vi "Load Cryostat Class.vi"(8 "error in (no error)":errorcluster, 11 "SweepControl in":refnum<class "SweepControl.lvclass">) -> (0 "error out":errorcluster, 3 "SweepControl out":refnum<class "SweepControl.lvclass">)   [LabVIEW 2016]
uses:
  <userlib>/LevyLab/Levylab Instruments/Instrument Types/Cryostat/Instrument.Cryostat.lvclass
  Control Experiment/Control Experiment.lvclass
  SweepControl.lvclass
  C:/Program Files (x86)/National Instruments/LabVIEW 2016/vi.lib/JKI/JKI SMO/SMO/SMO.lvclass
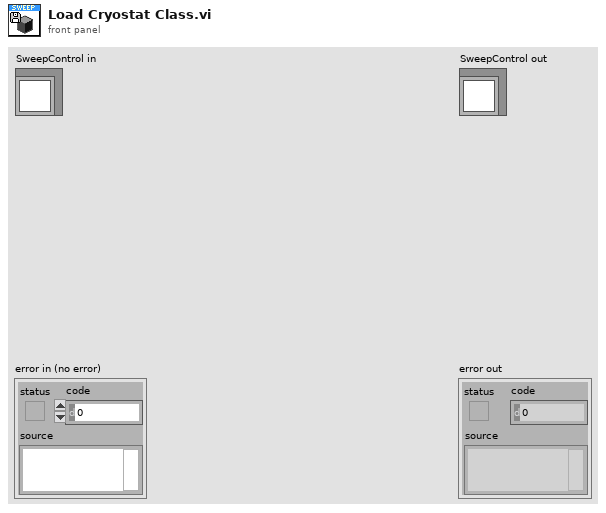
[diagram p1: front panel]
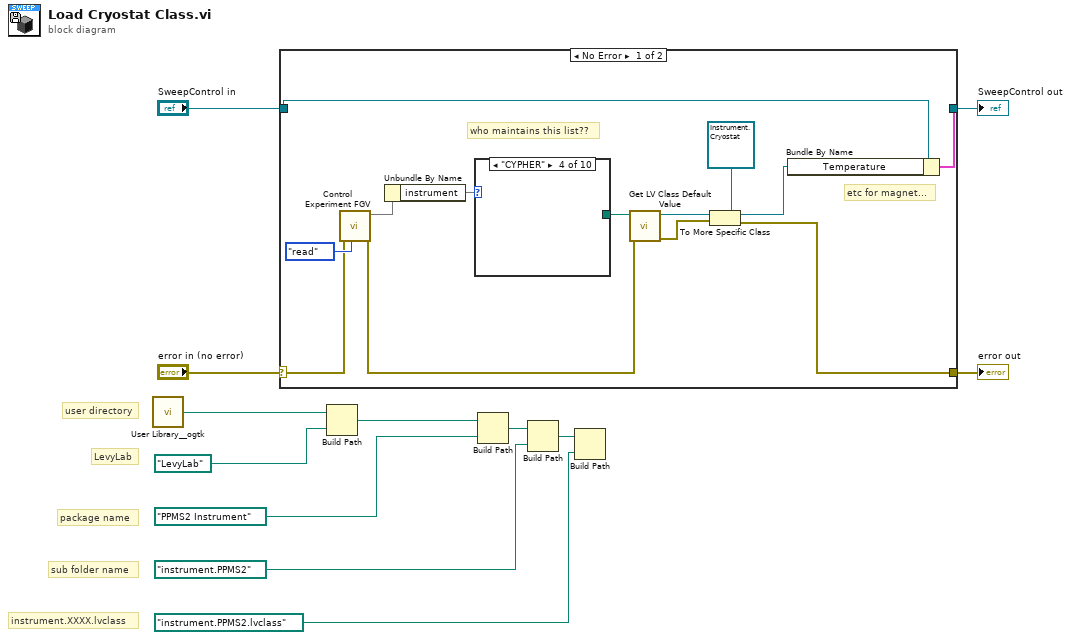
[diagram p0: block diagram]
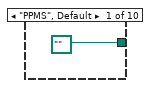
[diagram p2: hidden frame]
diagram:
  # "LevyLab"
  # "user directory"
  # "instrument.XXXX.lvclass"
  # "sub folder name"
  # "package name"
  n1 = call <userlib>:"User Library__ogtk.vi"() -> ("User Library (+ Relative)"=w8:path)  [unwired: 1 in]
  n2 = case shown="No Error" "error in (no error)" {
    selector: "error in (no error)" -> [w17 w28]
    tunnel: [w20 w28] -> w11
    tunnel: [w21 w27] -> w9
    tunnel: "SweepControl in" -> [w22 w27]
    frame No Error {
      # "who maintains this list??"
      # "etc for magnet..."
      n3 = call "Control Experiment FGV.vi"("Function"=enum16{"read", "write"}."read", "error in (no error)"=w17) -> ("error out"=w16:errorcluster, 2:w13)  [unwired: 7 in, 1 out]
      n4 = Unbundle By Name(w13) -> ("instrument"=w15)
      n5 = case shown="\"CYPHER\"" w15 {
        tunnel: [path "" ("class path") _ _ _ _ _ _ _ _ _] -> w14
        frame "PPMS", Default {
        }
        frame "PPMS2" {
        }
        frame "MFP3D" {
        }
        frame "CYPHER" {
        }
        frame "THz1" {
        }
        frame "THz2" {
        }
        frame "MNK" {
        }
        frame "CF900" {
        }
        frame "JEOL" {
        }
        frame "AGILENT" {
        }
      }
      n6 = call <vilib>:"Get LV Class Default Value.vi"("error in (no error)"=w16, "class path"=w14) -> ("error out"=w24:errorcluster, "object"=w23:refnum<class>)  [unwired: 8 in]
      n7 = To More Specific Class(target class=refnum<class "Instrument.Cryostat.lvclass"> refnum ("Instrument.Cryostat in"), reference=w23, error in=w24) -> (specific class reference=w19:refnum<class "Instrument.Cryostat.lvclass">, error out=w20:errorcluster)
      n8 = Bundle By Name(cluster=w22, "Temperature"=w19) -> (w21:cluster{})
    }
    frame Error {
    }
  }
  "error out" <- w11
  "SweepControl out" <- w9
  n9 = Build Path(base path=w8, name or relative path=path "LevyLab" ("class path")) -> (appended path=w7:path)
  n10 = Build Path(base path=w7, name or relative path=path "PPMS2 Instrument" ("class path")) -> (appended path=w6:path)
  n11 = Build Path(base path=w6, name or relative path=path "instrument.PPMS2" ("class path")) -> (appended path=w5:path)
  n12 = Build Path(base path=w5, name or relative path=path "instrument.PPMS2.lvclass" ("class path")) -> ()  [unwired: 1 out]
